vi "Begin.vi"() -> (0 "error out":errorcluster)   [LabVIEW 2013]
doc: "Called before other user functions, this VI is expected to open initial I/O refnums, load in file data, and do all program initialization. Notice that the <B>error out</B> terminal is simply used for data flow. Wiring it to other structures or subVIs ensures that this VI runs first."
uses:
  <vilib>/Rock Robotics/WPI/SafetyOutput/WPI_SafetyOutputConfigMenu.ctl
  <vilib>/Rock Robotics/WPI/DriverStation/WPI_DriverStationRobotMode2.ctl
  <vilib>/Rock Robotics/WPI/Joystick/WPI_JoystickDeviceEnum.ctl
  <vilib>/Rock Robotics/SystemInterfaces/DIO/FPGA_DIOChannel.ctl
  <vilib>/Rock Robotics/WPI/Solenoid/WPI_SolenoidChannel.ctl
  <vilib>/Rock Robotics/SystemInterfaces/AI/FPGA_AIChannel.ctl
  Robot Global Data.vi
  <vilib>/Rock Robotics/WPI/Counter/WPI_CounterDigitalInputToDigitalSource.vi
  <vilib>/Rock Robotics/WPI/Solenoid/WPI_SolenoidOpenDouble.vi
  <vilib>/Rock Robotics/WPI/RobotDrive/WPI_RobotDriveOpen4MotorWithCANJaguar.vi
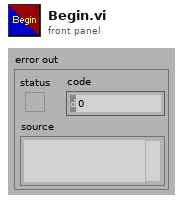
[diagram p1: front panel]
types:
  T1 = typedef "FPGA_AIChannel.ctl" = enum8{"AI 1", "AI 2", "AI 3", "AI 4", "AI 5", "AI 6", "AI 7", "AI 8", "Invalid"}
  T2 = typedef "WPI_SolenoidChannel.ctl" = enum8{"Solenoid 1", "Solenoid 2", "Solenoid 3", "Solenoid 4", "Solenoid 5", "Solenoid 6", "Solenoid 7", "Solenoid 8", "Invalid"}
  T3 = typedef "FPGA_DIOChannel.ctl" = enum8{"DIO 1", "DIO 2", "DIO 3", "DIO 4", "DIO 5", "DIO 6", "DIO 7", "DIO 8", "DIO 9", "DIO 10", "DIO 11", "DIO 12", "DIO 13", "DIO 14", "Invalid"}
  T4 = typedef "WPI_JoystickDeviceEnum.ctl" = enum16{"USB 1", "USB 2", "USB 3", "USB 4", "Kinect 1", "Kinect 2"}
  T5 = typedef "WPI_DriverStationRobotMode2.ctl" = enum16{"Autonomous Disabled", "Autonomous Enabled", "Teleop Disabled", "Teleop Enabled", "Timeout", "Finish", "Test Disabled", "Test Enabled"}
  T6 = typedef "WPI_SafetyOutputConfigMenu.ctl" = enum16{"Enable", "Disable"}
  T7 = typedef "WPI_DigitalInputDevRef.ctl" = cluster{"DevStatus":errorcluster, "DIO Channel":T3, "Digital Module":T8}
  T8 = typedef "FPGA_TypedefDigitalModule.ctl" = enum16{"Digital Module 1", "Digital Module 2"}
  T9 = typedef "WPI_AnalogChannelDevRef.ctl" = cluster{"DevStatus":errorcluster, "Analog Module":T10, "Analog Channel":T1}
  T10 = typedef "FPGA_TypedefAnalogModule.ctl" = enum16{"Analog Module 1", "Analog Module 2"}
  T11 = typedef "FPGA_CounterEncoderSourceConvertionLVSourceType.ctl" = cluster{"DevStatus":errorcluster, "AnalogTriggerMode?":bool, "DigitalMode":cluster{"Digital Module":T8, "DIO Channel":T12}, "AnalogTriggerMode":cluster{"AnalogTriggerIndex":T13, "OutputType":T14}}
  T12 = typedef "FPGA_DIODigitalSourceChannel.ctl" = enum8{"DIO 1", "DIO 2", "DIO 3", "DIO 4", "DIO 5", "DIO 6", "DIO 7", "DIO 8", "DIO 9", "DIO 10", "DIO 11", "DIO 12", "DIO 13", "DIO 14", "Disabled"}
  T13 = typedef "FPGA_AnalogTriggerIndex.ctl" = enum8{"Trig 0", "Trig 1", "Trig 2", "Trig 3", "Trig 4", "Trig 5", "Trig 6", "Trig 7", "Invalid"}
  T14 = typedef "FPGA_AnalogTriggerOutType.ctl" = enum16{"InWindow", "TriggerState", "Rising", "Falling"}
  T15 = typedef "WPI_RobotDriveDevRef.ctl" = cluster{"DevStatus":errorcluster, "Motors[]":T16[], "Square Inputs":bool, "Max Output":dbl, "Isochronous":bool}
  T16 = typedef "WPI_MotorControlDeviceRef.ctl" = cluster{"DeviceStatus":errorcluster, "Type":enum16{"PWM", "CAN"}, "PWM":cluster{"Digital Module":T8, "PWM Channel":T17, "DeadBand":T18}, "CAN":cluster{"Device Number":u8, "Control Mode":T19, "Semaphore":T20, "Max Vout":dbl}, "Invert":bool, "TransformRef":T21, "InvTransformRef":T21}
  T17 = typedef "FPGA_DIOPWMChannel.ctl" = enum8{"PWM 1", "PWM 2", "PWM 3", "PWM 4", "PWM 5", "PWM 6", "PWM 7", "PWM 8", "PWM 9", "PWM 10", "Invalid"}
  T18 = typedef "WPI_PWMDeadband.ctl" = cluster{"Name":string, "maxPositivePwm":i32, "minPositivePwm":i32, "centerPwm":i32, "maxNegativePwm":i32, "minNegativePwm":i32, "angularRange":u16}
  T19 = typedef "WPI_CANJaguar_ControlMode.ctl" = enum8{"Percent VBus", "Current", "Speed", "Position", "Voltage"}
  T20 = typedef "Semaphore RefNum" = refnum<k1>
  T21 = typedef "WPI_PWMTransform_ConPane.ctl" = refnum<vi>
  T22 = typedef "WPI_EncoderDevRef.ctl" = cluster{"DevStatus":errorcluster, "EncoderIndex":T23, "CounterIndex":T24, "DistancePerCount":dbl, "Decoding Type":T25}
  T23 = typedef "FPGA_EncoderIdx.ctl" = enum8{"Enc 0", "Enc 1", "Enc 2", "Enc 3", "Invalid"}
  T24 = typedef "FPGA_CounterCtrSystemIndex.ctl" = enum8{"Ctr 0", "Ctr 1", "Ctr 2", "Ctr 3", "Ctr 4", "Ctr 5", "Ctr 6", "Ctr 7", "Invalid"}
  T25 = typedef "WPI_EncoderType.ctl" = enum16{"1x", "2x", "4x"}
  T26 = typedef "WPI_JoystickDevRef.ctl" = cluster{"Device":T4}
  T27 = typedef "WPI_SolenoidDevRef.ctl" = cluster{"DevStatus":errorcluster, "Solenoid Module":T28, "Forward Solenoid Channel":T2, "Reverse Solenoid Channel":T2}
  T28 = typedef "FPGA_TypedefSolenoidModule.ctl" = enum16{"Solenoid Module 1", "Solenoid Module 2"}
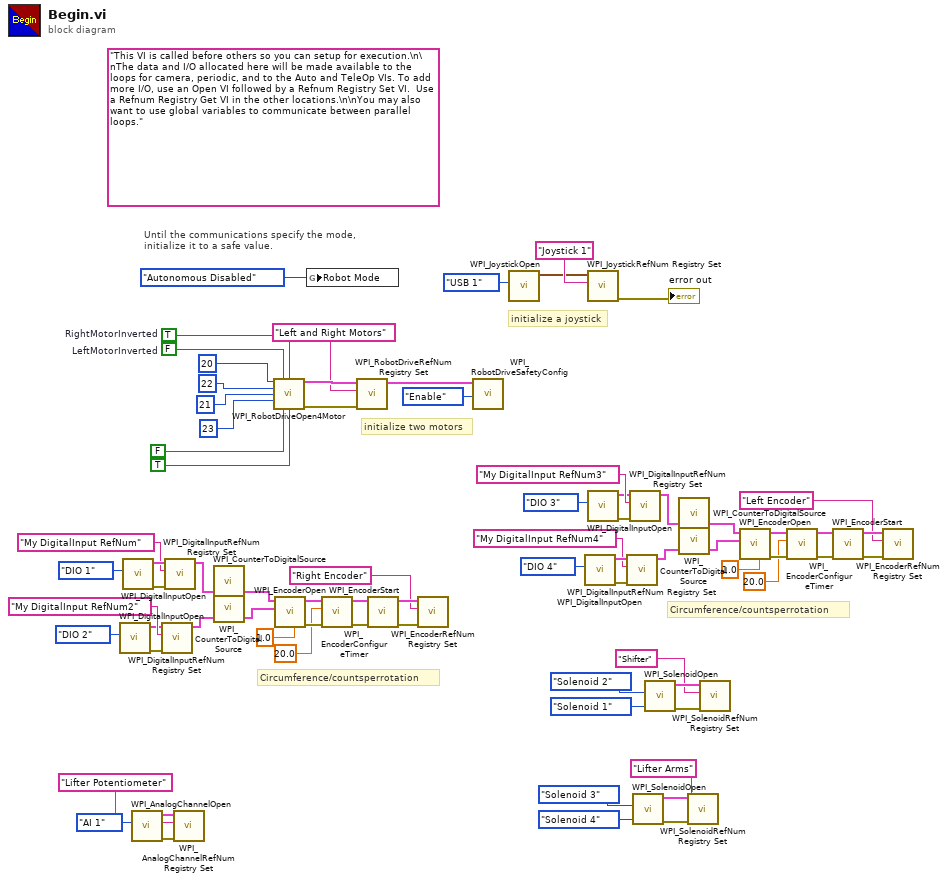
[diagram p0: block diagram]
diagram:
  (unwired) "This VI is called before others so you can setup for execution.\n\nThe data and I/O allocated here will be made available to the loops for camera, periodic, and to the Auto and TeleOp VIs. To add more I/O, use an Open VI followed by a Refnum Registry Set VI.  Use a Refnum Registry Get VI in the other locations.\n\nYou may also want to use global variables to communicate between parallel loops."
  w14 = FALSE  # LeftMotorInverted
  w13 = TRUE  # RightMotorInverted
  # "Circumference/countsperrotation"
  # "Circumference/countsperrotation"
  # "initialize a joystick"
  # "Until the communications specify the mode,\ninitialize it to a safe value."
  # "initialize two motors"
  n1 = call <vilib>:"WPI_DigitalInputOpen.vi"("DIO Channel"=FPGA_DIOChannel."DIO 2") -> ("error out"=w45:errorcluster, "DigitalInputDevRef"=w46:T7)  [unwired: 9 in]
  n2 = call <vilib>:"WPI_DigitalInputOpen.vi"("DIO Channel"=FPGA_DIOChannel."DIO 1") -> ("error out"=w54:errorcluster, "DigitalInputDevRef"=w53:T7)  [unwired: 9 in]
  n3 = call <vilib>:"WPI_AnalogChannelOpen.vi"("Analog Channel"=FPGA_AIChannel."AI 1") -> ("error out"=w4:errorcluster, "AIDeviceRef"=w3:T9)  [unwired: 9 in]
  n4 = call <vilib>:"WPI_DigitalInputRefNum Registry Set.vi"("error in (no error)"=w45, "refnum name"="My DigitalInput RefNum2", "DigitalInputDevRef"=w46) -> ("DigitalInputDevRef"=w44:T7)  [unwired: 7 in, 1 out]
  n5 = call <vilib>:"WPI_DigitalInputRefNum Registry Set.vi"("error in (no error)"=w54, "refnum name"="My DigitalInput RefNum", "DigitalInputDevRef"=w53) -> ("DigitalInputDevRef"=w52:T7)  [unwired: 7 in, 1 out]
  n6 = call <vilib>:"WPI_AnalogChannelRefNum Registry Set.vi"("error in (no error)"=w4, "refnum name"="Lifter Potentiometer", "AIDeviceRef"=w3) -> ()  [unwired: 7 in, 2 out]
  n7 = call-poly <vilib>:"WPI_CounterToDigitalSource.vi"("DigitalInputDevRef"=w52) -> ("Digital Source"=w55:T11)  [unwired: 6 in]
  n8 = call-poly <vilib>:"WPI_CounterToDigitalSource.vi"("DigitalInputDevRef"=w44) -> ("Digital Source"=w50:T11)  [unwired: 6 in]
  n9 = call-poly <vilib>:"WPI_RobotDriveOpen4Motor.vi"("Rear Left Motor"=u8 20, "Rear Left Motor Inverted"=w14, "Rear Right Motor Inverted"=w13, "Rear Right Motor"=u8 22, "Front Left Motor"=u8 21, "Front Right Motor"=u8 23, "Front Left Motor Inverted"=FALSE, "Front Right Motor Inverted"=TRUE) -> ("RobotDriveDevRef"=w74:T15, "error out"=w72:errorcluster)  [unwired: 6 in]
  n10 = call <vilib>:"WPI_EncoderOpen.vi"("DistancePerCount"=1.0, "BSource"=w50, "ASource"=w55) -> ("error out"=w61:errorcluster, "EncoderDevRef"=w60:T22)  [unwired: 7 in]
  n11 = global write "Robot Global Data.vi" "Robot Mode"(WPI_DriverStationRobotMode2."Autonomous Disabled" ("Robot Mode")) -> ()
  n12 = call <vilib>:"WPI_EncoderConfigureTimer.vi"("error in (no error)"=w61, "Minimum Rate"=20.0, "EncoderDevRef"=w60) -> ("error out"=w59:errorcluster, "EncoderDevRef"=w58:T22)  [unwired: 7 in]
  n13 = call <vilib>:"WPI_RobotDriveRefNum Registry Set.vi"("error in (no error)"=w72, "refnum name"="Left and Right Motors", "RobotDriveDevRef"=w74) -> ("RobotDriveDevRef"=w71:T15)  [unwired: 8 out]
  n14 = call <vilib>:"WPI_EncoderStart.vi"("error in (no error)"=w59, "EncoderDevRef"=w58) -> ("error out"=w57:errorcluster, "EncoderDevRef"=w56:T22)  [unwired: 8 in]
  n15 = call <vilib>:"WPI_EncoderRefNum Registry Set.vi"("error in (no error)"=w57, "refnum name"="Right Encoder", "EncoderDevRef"=w56) -> ()  [unwired: 7 in, 2 out]
  n16 = call <vilib>:"WPI_RobotDriveSafetyConfig.vi"("mode"=WPI_SafetyOutputConfigMenu."Enable", "RobotDriveDevRef"=w71) -> ()  [unwired: 8 in, 2 out]
  n17 = call <vilib>:"WPI_JoystickOpen.vi"("JoystickDevice"=WPI_JoystickDeviceEnum."USB 1") -> ("JoystickDevRef"=w67:T26)  [unwired: 10 in]
  n18 = call <vilib>:"WPI_DigitalInputOpen.vi"("DIO Channel"=FPGA_DIOChannel."DIO 4") -> ("error out"=w40:errorcluster, "DigitalInputDevRef"=w39:T7)  [unwired: 9 in]
  n19 = call <vilib>:"WPI_JoystickRefNum Registry Set.vi"("refnum name"="Joystick 1", "JoystickDevRef"=w67) -> ("error out"=→"error out":errorcluster)  [unwired: 8 in, 1 out]
  n20 = call <vilib>:"WPI_DigitalInputOpen.vi"("DIO Channel"=FPGA_DIOChannel."DIO 3") -> ("error out"=w31:errorcluster, "DigitalInputDevRef"=w32:T7)  [unwired: 9 in]
  n21 = call <vilib>:"WPI_DigitalInputRefNum Registry Set.vi"("error in (no error)"=w40, "refnum name"="My DigitalInput RefNum4", "DigitalInputDevRef"=w39) -> ("DigitalInputDevRef"=w41:T7)  [unwired: 7 in, 1 out]
  n22 = call <vilib>:"WPI_DigitalInputRefNum Registry Set.vi"("error in (no error)"=w31, "refnum name"="My DigitalInput RefNum3", "DigitalInputDevRef"=w32) -> ("DigitalInputDevRef"=w33:T7)  [unwired: 7 in, 1 out]
  n23 = call-poly <vilib>:"WPI_SolenoidOpen.vi"("Reverse Solenoid Channel"=WPI_SolenoidChannel."Solenoid 4", "Forward Solenoid Channel"=WPI_SolenoidChannel."Solenoid 3") -> ("error out"=w6:errorcluster, "SolenoidDevRef"=w7:T27)  [unwired: 8 in]
  n24 = call-poly <vilib>:"WPI_SolenoidOpen.vi"("Reverse Solenoid Channel"=WPI_SolenoidChannel."Solenoid 1", "Forward Solenoid Channel"=WPI_SolenoidChannel."Solenoid 2") -> ("error out"=w19:errorcluster, "SolenoidDevRef"=w18:T27)  [unwired: 8 in]
  n25 = call-poly <vilib>:"WPI_CounterToDigitalSource.vi"("DigitalInputDevRef"=w33) -> ("Digital Source"=w30:T11)  [unwired: 6 in]
  n26 = call-poly <vilib>:"WPI_CounterToDigitalSource.vi"("DigitalInputDevRef"=w41) -> ("Digital Source"=w35:T11)  [unwired: 6 in]
  n27 = call <vilib>:"WPI_SolenoidRefNum Registry Set.vi"("error in (no error)"=w6, "refnum name"="Lifter Arms", "SolenoidDevRef"=w7) -> ()  [unwired: 7 in, 2 out]
  n28 = call <vilib>:"WPI_SolenoidRefNum Registry Set.vi"("error in (no error)"=w19, "refnum name"="Shifter", "SolenoidDevRef"=w18) -> ()  [unwired: 7 in, 2 out]
  n29 = call <vilib>:"WPI_EncoderOpen.vi"("DistancePerCount"=1.0, "BSource"=w35, "ASource"=w30) -> ("error out"=w24:errorcluster, "EncoderDevRef"=w25:T22)  [unwired: 7 in]
  n30 = call <vilib>:"WPI_EncoderConfigureTimer.vi"("error in (no error)"=w24, "Minimum Rate"=20.0, "EncoderDevRef"=w25) -> ("error out"=w26:errorcluster, "EncoderDevRef"=w27:T22)  [unwired: 7 in]
  n31 = call <vilib>:"WPI_EncoderStart.vi"("error in (no error)"=w26, "EncoderDevRef"=w27) -> ("error out"=w28:errorcluster, "EncoderDevRef"=w29:T22)  [unwired: 8 in]
  n32 = call <vilib>:"WPI_EncoderRefNum Registry Set.vi"("error in (no error)"=w28, "refnum name"="Left Encoder", "EncoderDevRef"=w29) -> ()  [unwired: 7 in, 2 out]
